vi "test-state-machine.vi"() -> ()   [LabVIEW 2019, in "test-state-machine.lvlib"]
uses:
  test-state-machine.lvlib
  ade17a7d-1626-4547-8189-477ef3731f16.vi
  Action Type.ctl
  Event Type.ctl
  Guard Type.ctl
  State Type.ctl
  246338fd-fa47-43ef-9d25-2d0435b74198.vi
  guards.vi
  actions.vi
  ce21debc-ef52-4a03-aab6-b5db00547d1d.vi
  State Data.ctl
panel:
  out "mermaid.js state diagram":string
  in  "previous":bool
  in  "next":bool
  in  "repeat mode":bool
  in  "error":bool
  in  "autoplay":bool
  in  "track done":bool
  out "state":T1
  in  "end pause":bool
  in  "pause":bool
  in  "cd_detected":bool
  in  "stop":bool
  in  "open_close":bool
  in  "play":bool
  out "state":T3=enum."Open"
  in  "initial state":T1={"auto play?"=FALSE, "good disc?"=TRUE, "last action"=enum."null action", "track #"=0, "# tracks"=0, "repeat"=enum."none"}
  out "error out":errorcluster
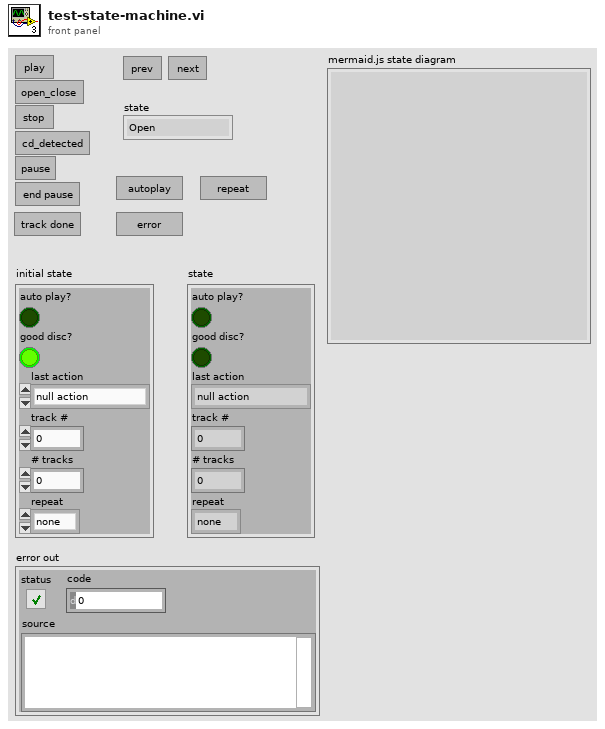
[diagram p1: front panel]
types:
  T1 = typedef "test-state-machine.lvlib/State Data.ctl" = cluster{"auto play?":bool, "good disc?":bool, "last action":T2, "track #":u8, "# tracks":u8, "repeat":enum16{"none", "one", "all"}}
  T2 = typedef "test-state-machine.lvlib/Action Type.ctl" = enum16{"null action", "start_playback", "open_drawer", "close_drawer", "store_cd_info", "stop_playback", "pause_playback", "stop_and_open", "resume_playback", "next_track", "prev_track", "repeat_track", "play_first", "toggle_autoplay", "stop_safe", "toggle_repeat_mode"}
  T3 = typedef "test-state-machine.lvlib/State Type.ctl" = enum16{"Stopped", "Open", "Empty", "Playing", "Paused", "Error"}
  T4 = typedef "test-state-machine.lvlib/Guard Type.ctl" = enum16{"auto_start", "good_disk_format", "has_next_track", "has_prev_track", "repeat_one", "last_track_and_repeat", "last_track"}
  T5 = typedef "test-state-machine.lvlib/Event Type.ctl" = enum16{"play", "open_close", "stop", "cd_detected", "pause", "end_pause", "track_done", "autoplay", "error", "repeat_mode", "next", "previous"}
  T6 = map{T3, map{T5, cluster{"State Type":T3, "Action Type":T2, bool, "Guard Type":T4, bool}[]}}
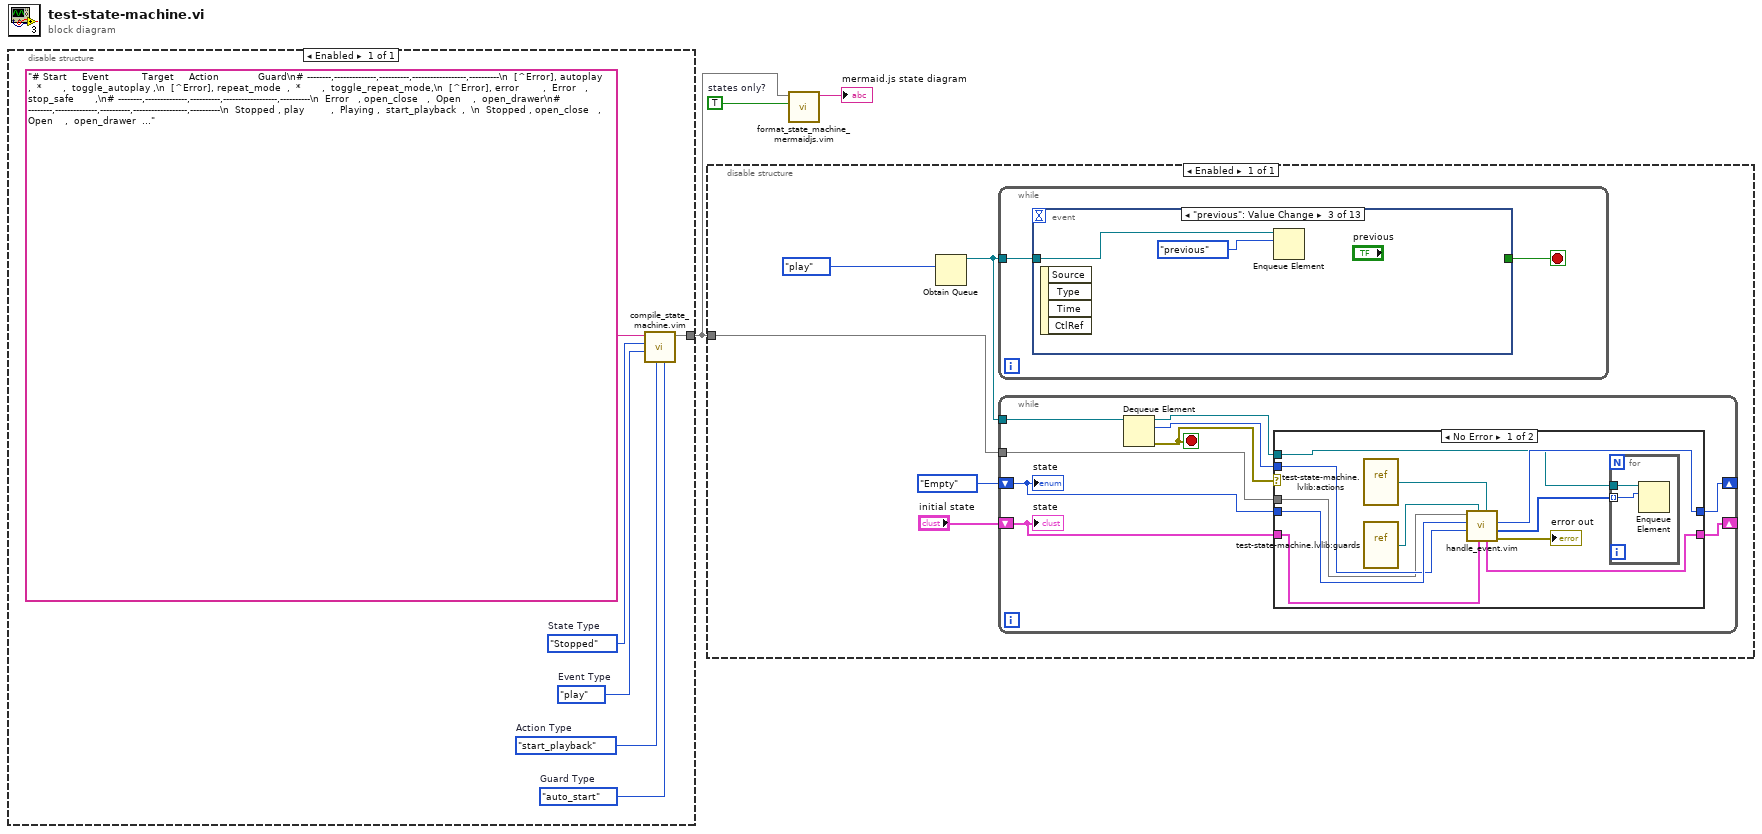
[diagram p0: block diagram]
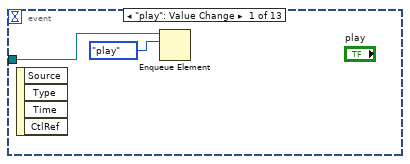
[diagram p3: hidden frame]
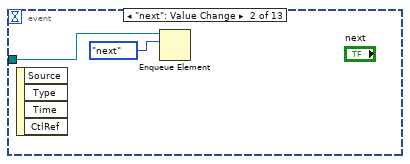
[diagram p4: hidden frame]
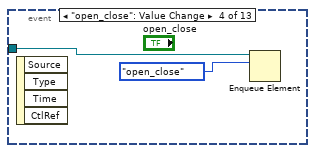
[diagram p5: hidden frame]
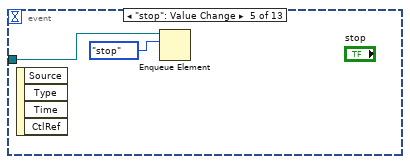
[diagram p6: hidden frame]
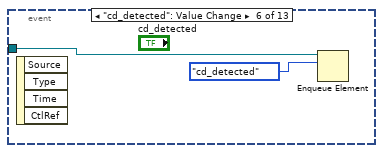
[diagram p7: hidden frame]
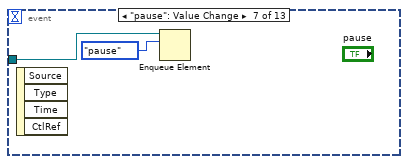
[diagram p8: hidden frame]
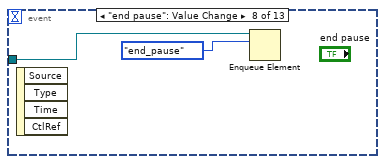
[diagram p9: hidden frame]
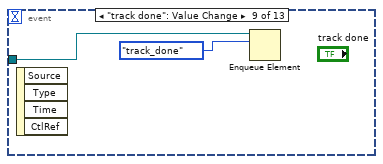
[diagram p10: hidden frame]
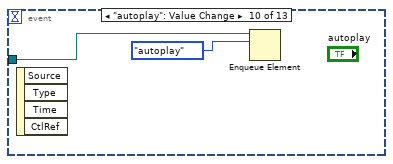
[diagram p11: hidden frame]
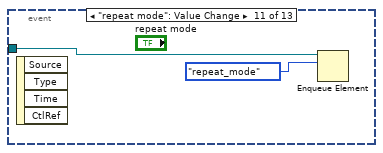
[diagram p12: hidden frame]
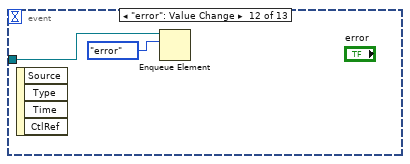
[diagram p13: hidden frame]
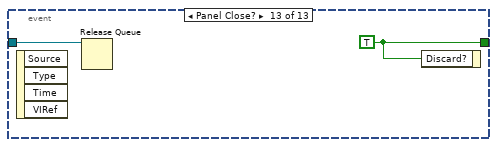
[diagram p14: hidden frame]
diagram:
  w1 = TRUE  # states only?
  n1 = disable-structure shown="Enabled" {
    disable-tunnel: [w4] -> w3
    frame Enabled {
      w8 = State_Type."Stopped"  # State Type
      w5 = Guard_Type."auto_start"  # Guard Type
      w7 = Event_Type."play"  # Event Type
      w6 = Action_Type."start_playback"  # Action Type
      n2 = call "compile_state_machine.vim"("Guard Type"=w5, "Action Type"=w6, "Event Type"=w7, "State Type"=w8, "state machine definition"="# Start     Event           Target     Action             Guard\n# --------,--------------,----------,------------------,----------\n  [^Error], autoplay     ,  *       ,  toggle_autoplay ,\n  [^Error], repeat_mode  ,  *       ,  toggle_repeat_mode,\n  [^Error], error        ,  Error   ,  stop_safe       ,\n# --------,--------------,----------,------------------,----------\n  Error   , open_close   ,  Open    ,  open_drawer\n# --------,--------------,----------,------------------,----------\n  Stopped , play         ,  Playing ,  start_playback  ,  \n  Stopped , open_close   ,  Open    ,  open_drawer     ,  \n  Stopped , stop         ,  Stopped ,                  ,\n# --------,--------------,----------,------------------,-----------\n  Open    , open_close   ,  Empty   ,  close_drawer    ,\n# --------,--------------,----------,------------------,-----------\n  Empty   , open_close   ,  Open    ,  open_drawer     ,\n  Empty   , cd_detected  ,  Playing ,  store_cd_info   ,  auto_start\n  Empty   , cd_detected  ,  Stopped ,  store_cd_info   ,  \n# --------,--------------,----------,------------------,-----------\n  Playing , stop         ,  Stopped ,  stop_playback   ,\n  Playing , pause        ,  Paused  ,  pause_playback  ,\n  Playing , open_close   ,  Open    ,  stop_and_open   ,\n  Playing , next         ,  Playing ,  play_first      , last_track_and_repeat\n  Playing , next         ,  Playing ,  next_track      , has_next_track\n  Playing , previous     ,  Playing ,  prev_track      , has_prev_track\n  Playing , track_done   ,  Playing ,  repeat_track    , repeat_one\n  Playing , track_done   ,  Playing ,  next_track      , has_next_track\n  Playing , track_done   ,  Playing ,  play_first      , last_track_and_repeat\n  Playing , track_done   ,  Stopped ,  stop_playback   , last_track\n# --------,--------------,----------,------------------,-----------\n  Paused  , end_pause    ,  Playing ,  resume_playback ,\n  Paused  , stop         ,  Stopped ,  stop_playback   ,\n  Paused  , open_close   ,  Open    ,  stop_and_open   ,\n  Paused  , play         ,  Playing ,  resume_playback , \n  Paused  , pause        ,  Playing ,  resume_playback ,") -> ("map"=w4:T6)  [unwired: 5 in, 1 out]
    }
  }
  n3 = disable-structure shown="Enabled" {
    disable-tunnel: w3 -> [w13]
    frame Enabled {
      n4 = Obtain Queue(element data type=Event_Type."play" ("Event Type")) -> (queue out=w12:refnum<queue>)  [unwired: 4 in, 2 out]
      n5 = while {
        tunnel: w12 -> [w39]
        stop <- w40 stop-if-true
        n6 = event shown="[2] \"previous\": Value Change" {
          selector: _ -> [_ _ _ _ _ _ _ _ _ _ _ _ _]
          dyn-events: _ -> [_ _ _ _ _ _ _ _ _ _ _ _ _]
          timeout: _ -> [_ _ _ _ _ _ _ _ _ _ _ _ _]
          tunnel: [_ _ _ _ _ _ _ _ _ _ _ _ w66] -> w40
          tunnel: w39 -> [w42 w44 w46 w48 w50 w52 w54 w56 w58 w60 w62 w64 w65]
          event "play": Value Change {
            n7 = event-data() -> ()  [unwired: 1 in, 4 out]
            n8 = Enqueue Element(queue=w42, element=Event_Type."play" ("Event Type")) -> ()  [unwired: 2 in, 3 out]
          }
          event "next": Value Change {
            n9 = event-data() -> ()  [unwired: 1 in, 4 out]
            n10 = Enqueue Element(queue=w44, element=Event_Type."next" ("Event Type")) -> ()  [unwired: 2 in, 3 out]
          }
          event "previous": Value Change {
            n11 = event-data() -> ()  [unwired: 1 in, 4 out]
            n12 = Enqueue Element(queue=w46, element=Event_Type."previous" ("Event Type")) -> ()  [unwired: 2 in, 3 out]
          }
          event "open_close": Value Change {
            n13 = event-data() -> ()  [unwired: 1 in, 4 out]
            n14 = Enqueue Element(queue=w48, element=Event_Type."open_close" ("Event Type")) -> ()  [unwired: 2 in, 3 out]
          }
          event "stop": Value Change {
            n15 = event-data() -> ()  [unwired: 1 in, 4 out]
            n16 = Enqueue Element(queue=w50, element=Event_Type."stop" ("Event Type")) -> ()  [unwired: 2 in, 3 out]
          }
          event "cd_detected": Value Change {
            n17 = event-data() -> ()  [unwired: 1 in, 4 out]
            n18 = Enqueue Element(queue=w52, element=Event_Type."cd_detected" ("Event Type")) -> ()  [unwired: 2 in, 3 out]
          }
          event "pause": Value Change {
            n19 = event-data() -> ()  [unwired: 1 in, 4 out]
            n20 = Enqueue Element(queue=w54, element=Event_Type."pause" ("Event Type")) -> ()  [unwired: 2 in, 3 out]
          }
          event "end pause": Value Change {
            n21 = event-data() -> ()  [unwired: 1 in, 4 out]
            n22 = Enqueue Element(queue=w56, element=Event_Type."end_pause" ("Event Type")) -> ()  [unwired: 2 in, 3 out]
          }
          event "track done": Value Change {
            n23 = event-data() -> ()  [unwired: 1 in, 4 out]
            n24 = Enqueue Element(queue=w58, element=Event_Type."track_done" ("Event Type")) -> ()  [unwired: 2 in, 3 out]
          }
          event "autoplay": Value Change {
            n25 = event-data() -> ()  [unwired: 1 in, 4 out]
            n26 = Enqueue Element(queue=w60, element=Event_Type."autoplay" ("Event Type")) -> ()  [unwired: 2 in, 3 out]
          }
          event "repeat mode": Value Change {
            n27 = event-data() -> ()  [unwired: 1 in, 4 out]
            n28 = Enqueue Element(queue=w62, element=Event_Type."repeat_mode" ("Event Type")) -> ()  [unwired: 2 in, 3 out]
          }
          event "error": Value Change {
            n29 = event-data() -> ()  [unwired: 1 in, 4 out]
            n30 = Enqueue Element(queue=w64, element=Event_Type."error" ("Event Type")) -> ()  [unwired: 2 in, 3 out]
          }
          event Panel Close? {
            w66 = TRUE ("Discard?")
            n31 = event-data() -> ()  [unwired: 1 in, 4 out]
            n32 = Release Queue(queue=w65) -> ()  [unwired: 2 in, 3 out]
            n33 = event-data("Discard?"=w66) -> ()  [unwired: 1 in, 1 out]
          }
        }
      }
      n34 = while {
        tunnel: w12 -> [w23]
        tunnel: w13 -> [w21]
        shift-right: [w18] -> _
        shift-left: State_Type."Empty" ("State Type") -> [w20]
        shift-right: [w16] -> _
        shift-left: "initial state" -> [w15]
        stop <- w22 stop-if-true
        n35 = Dequeue Element(queue=w23) -> (queue out=w17:refnum<queue>, element=w19:T5, error out=w22:errorcluster)  [unwired: 2 in, 1 out]
        n36 = case shown="No Error" w22 {
          tunnel: w21 -> [w32 _]
          tunnel: w20 -> [w34 w38]
          tunnel: w19 -> [w33 _]
          tunnel: [w30 w38] -> w18
          tunnel: w17 -> [w27 _]
          tunnel: w15 -> [w25 w37]
          tunnel: [w24 w37] -> w16
          frame No Error {
            n37 = vi-ref "test-state-machine.lvlib:actions.vi"() -> (w28:refnum<vi>)
            n38 = vi-ref "test-state-machine.lvlib:guards.vi"() -> (w31:refnum<vi>)
            n39 = call "handle_event.vim"("actions"=w28, "state data in"=w25, "guards"=w31, "event"=w33, "state in"=w34, "map"=w32) -> ("error out"=→"error out":errorcluster, "events out"=w26:T5[], "state out"=w30:T3, "state data out"=w24:T1)  [unwired: 2 in]
            n40 = for {
              tunnel: w27 -> [w36]
              tunnel: w26 -> [w35] mode=indexing
              n41 = Enqueue Element(queue=w36, element=w35) -> ()  [unwired: 2 in, 3 out]
            }
          }
          frame Error {
          }
        }
        "state" <- w20
        "state" <- w15
      }
    }
  }
  n42 = call "format_state_machine_mermaidjs.vim"("states only?"=w1, "map"=w3) -> ("mermaidjs state machine"=→"mermaid.js state diagram":string)  [unwired: 9 in]
